vi "p4.4.vi"() -> ()   [LabVIEW 2020]
uses:
  <vilib>/Analysis/2dsp.llb/Upsample (DBL).vi
  <vilib>/Analysis/NI_AALBase.lvlib
  <vilib>/Analysis/NI_AALPro.lvlib
panel:
  in  "L = 2":i32=1
  in  "fs AD (Hz)":dbl=50000.0 min=0.0 max=50000.0
  in  "fs DA (Hz)":dbl=-1.0 min=-1.0 max=50000.0
  in  "Canal AD":tag="myDAQ1/audioInputLeft"
  in  "Canal DA":tag="myDAQ1/audioOutputLeft"
  out "error out":errorcluster
  out "Tono 3kHz":dbl[](graph)
  in  "Freq. tono":dbl=0.0078125 format="%0.4e"
  in  "Número muestras READ AD":i32
  in  "stop":bool
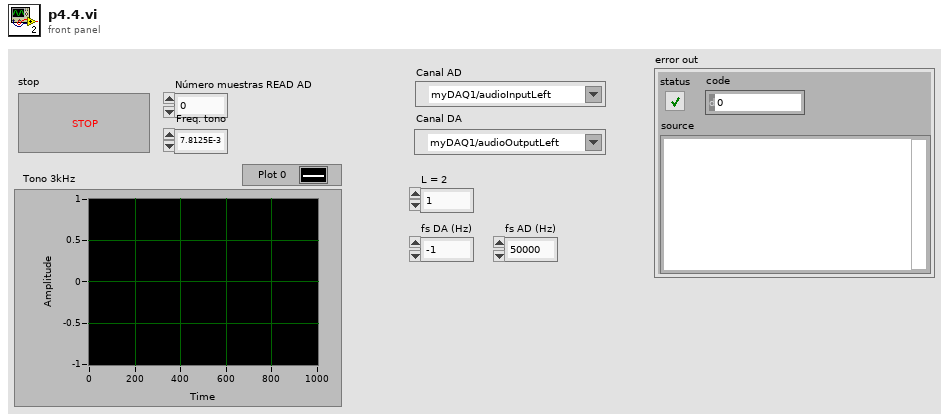
[diagram p1: front panel]
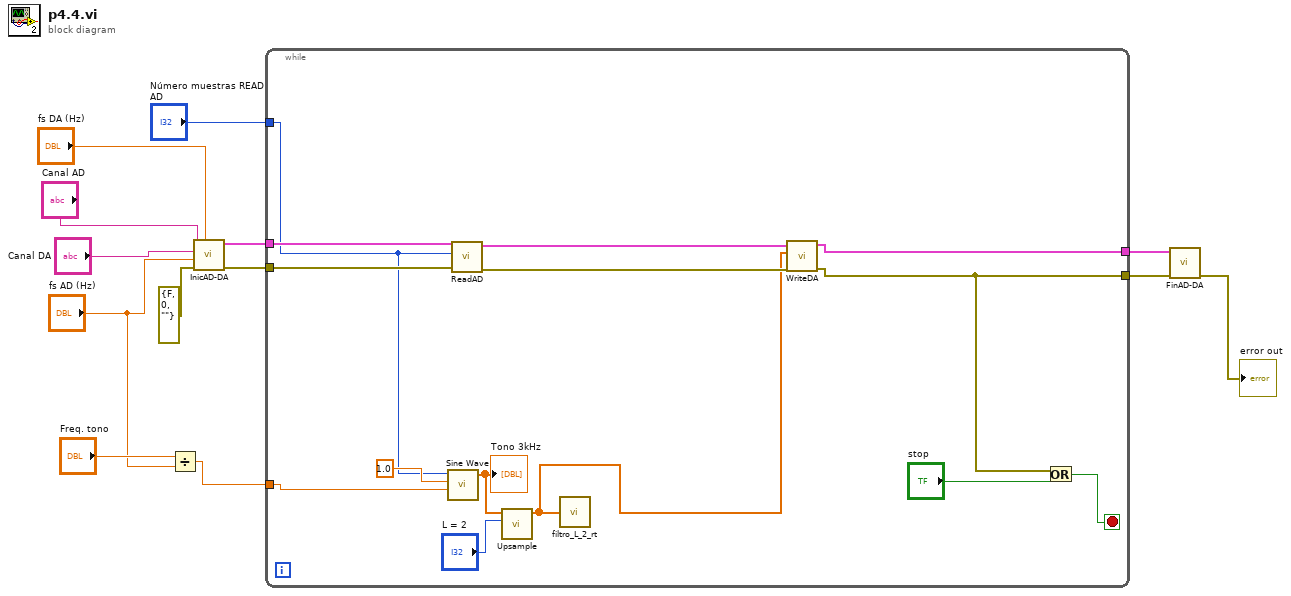
[diagram p0: block diagram]
diagram:
  n1 = Divide(x="Freq. tono", y="fs AD (Hz)") -> (x/y=w4:dbl)
  n2 = call <userlib>:"InicAD-DA.vi"("fs DA (Hz)"="fs DA (Hz)", "error in"=errorcluster {"status"=FALSE, "code"=0, "source"=""}, "fs AD (Hz)"="fs AD (Hz)", "Canal DA"="Canal DA", "Canal AD"="Canal AD") -> ("error out"=w10:errorcluster, "Tarea Out"=w11:cluster{"AD":refnum<k21>, "DA":refnum<k21>})  [unwired: 5 in]
  n3 = while {
    tunnel: [w26] -> w12
    tunnel: w11 -> [w25]
    tunnel: w10 -> [w24]
    tunnel: [w21] -> w9
    tunnel: "Número muestras READ AD" -> [w18]
    tunnel: w4 -> [w17]
    stop <- w22 stop-if-true
    n4 = call <vilib>:"Sine Wave.vi"("samples"=w18, "amplitude"=1.0, "frequency"=w17) -> ("sine wave"=w15:dbl[])  [unwired: 2 in, 2 out]
    "Tono 3kHz" <- w15
    n5 = call <userlib>:"ReadAD.vi"("error in"=w24, "numero de muestras"=w18, "Tarea In"=w25) -> ("error out"=w23:errorcluster, "Tarea Out"=w27:cluster{"AD":refnum<k21>, "DA":refnum<k21>})  [unwired: 6 in, 1 out]
    n6 = call-poly <vilib>:"Upsample.vi"("upsampling factor"="L = 2", "X"=w15) -> ("Upsampled Array"=w14:dbl[])  [unwired: 8 in, 1 out]
    n7 = call "filtro_L_2_rt.vi"("x"=w14) -> ()  [unwired: 1 out]
    n8 = call <userlib>:"WriteDA.vi"("error in"=w23, "Datos"=w14, "Tarea In"=w27) -> ("error out"=w21:errorcluster, "Tarea Out"=w26:cluster{"AD":refnum<k21>, "DA":refnum<k21>})  [unwired: 7 in]
    n9 = Or(x=w21, y="stop") -> (x .or. y?=w22:bool)
  }
  n10 = call <userlib>:"FinAD-DA.vi"("error in"=w9, "Tarea In"=w12) -> ("error out"=→"error out":errorcluster)  [unwired: 9 in]
